vi "testRotAng.vi"(8 "error in (no error)":errorcluster) -> (0 "error out":errorcluster)   [LabVIEW 2016]
doc: "Test to set/ get camera rotation angle in degree."
uses:
  CamRot/CamRot.lvclass
  <vilib>/addons/_JKI Toolkits/Caraya/classes/Test/Test.lvclass
  <vilib>/addons/_JKI Toolkits/Caraya/classes/Assert/Assert.lvclass
panel:
  in  "CamRot.lvclass":refnum<class "CamRot.lvclass">
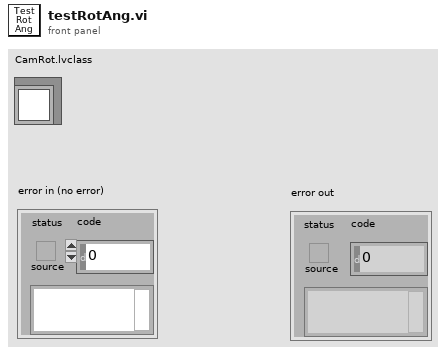
[diagram p1: front panel]
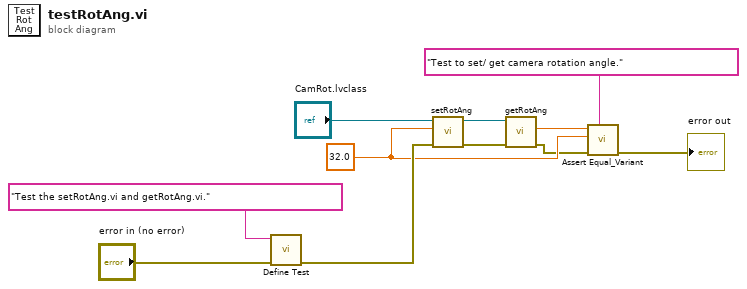
[diagram p0: block diagram]
diagram:
  w4 = 32.0 ("Rotation Angle in Deg")
  n1 = call <vilib>:"Define Test.vi"("error in (no error)"="error in (no error)", "Label (VI Title)"="Test the setRotAng.vi and getRotAng.vi.") -> ("error out"=w8:errorcluster)  [unwired: 9 in]
  n2 = call "setRotAng.vi"("error in (no error)"=w8, "Rotation Angle in Deg"=w4, "CamRot in"="CamRot.lvclass") -> ("error out"=w6:errorcluster, "CamRot out"=w7:refnum<class "CamRot.lvclass">)  [unwired: 7 in]
  n3 = call "getRotAng.vi"("error in (no error)"=w6, "CamRot in"=w7) -> ("error out"=w3:errorcluster, "Rotation Angle in Deg"=w5:dbl)  [unwired: 7 in, 1 out]
  n4 = call <vilib>:"Assert Equal_Variant.vi"("Label"="Test to set/ get camera rotation angle." ("Label (VI Title)"), "error in (no error)"=w3, "Y"=w4, "X"=w5) -> ("error out"=→"error out":errorcluster)  [unwired: 7 in]
